vi "Initialize.vi"(8 "error in (no error)":errorcluster, 11 "TelFocus in":refnum<class "TelFocus.lvclass">) -> (0 "error out":errorcluster, 3 "TelFocus out":refnum<class "TelFocus.lvclass">)   [LabVIEW 2018, in "TelFocus.lvclass"]
uses:
  TelFocus.lvclass
  Server/Server.lvclass
  Comm/Stream/Stream.lvclass
  Log/Log.lvclass
  SecMirror/SecMirror.lvclass
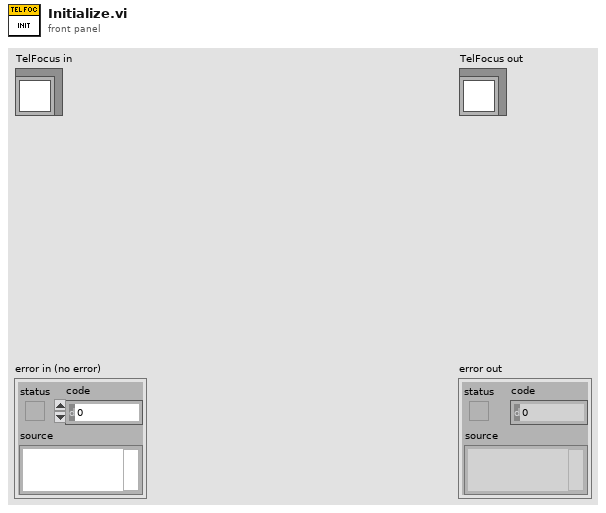
[diagram p1: front panel]
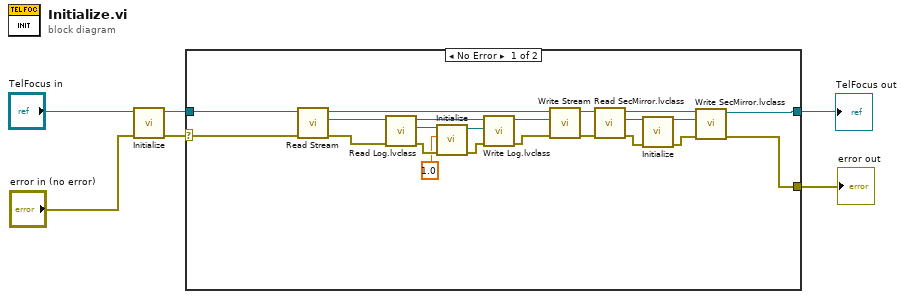
[diagram p0: block diagram]
diagram:
  n1 = call-parent "Initialize.vi"("error in (no error)"="error in (no error)", "Server in"="TelFocus in") -> ("error out"=w3:errorcluster, "Server out"=w4:refnum<class "TelFocus.lvclass">)  [unwired: 8 in]
  n2 = case shown="No Error" w3 {
    selector: w3 -> [w18 w29]
    tunnel: w4 -> [w19 w30]
    tunnel: [w9 w30] -> w2
    tunnel: [w10 w29] -> w1
    frame No Error {
      n3 = call-dynamic "Read Stream.vi"("error in (no error)"=w18, "Server in"=w19) -> ("error out"=w7:errorcluster, "Stream.lvclass"=w8:refnum<class "Stream.lvclass">, "Server out"=w28:refnum<class "TelFocus.lvclass">)  [unwired: 7 in]
      n4 = call-dynamic "Read Log.lvclass.vi"("error in (no error)"=w7, "Comm in"=w8) -> ("error out"=w24:errorcluster, "Log.lvclass"=w26:refnum<class "Log.lvclass">, "Comm out"=w27:refnum<class "Stream.lvclass">)  [unwired: 7 in]
      n5 = call-dynamic "Initialize.vi"("error in (no error)"=w24, "Level"=1.0, "Log in"=w26) -> ("error out"=w23:errorcluster, "Log out"=w25:refnum<class "Log.lvclass">)  [unwired: 7 in]
      n6 = call-dynamic "Write Log.lvclass.vi"("error in (no error)"=w23, "Log.lvclass"=w25, "Comm in"=w27) -> ("error out"=w21:errorcluster, "Comm out"=w22:refnum<class "Stream.lvclass">)  [unwired: 7 in]
      n7 = call-dynamic "Write Stream.vi"("error in (no error)"=w21, "Stream.lvclass"=w22, "Server in"=w28) -> ("error out"=w16:errorcluster, "Server out"=w17:refnum<class "TelFocus.lvclass">)  [unwired: 7 in]
      n8 = call-dynamic "Read SecMirror.lvclass.vi"("error in (no error)"=w16, "TelFocus in"=w17) -> ("error out"=w12:errorcluster, "SecMirror.lvclass"=w15:refnum<class "SecMirror.lvclass">, "TelFocus out"=w13:refnum<class "TelFocus.lvclass">)  [unwired: 7 in]
      n9 = call-dynamic "Initialize.vi"("error in (no error)"=w12, "SecMirror in"=w15) -> ("error out"=w11:errorcluster, "SecMirror out"=w14:refnum<class "SecMirror.lvclass">)  [unwired: 8 in]
      n10 = call-dynamic "Write SecMirror.lvclass.vi"("error in (no error)"=w11, "SecMirror.lvclass"=w14, "TelFocus in"=w13) -> ("error out"=w10:errorcluster, "TelFocus out"=w9:refnum<class "TelFocus.lvclass">)  [unwired: 7 in]
    }
    frame Error {
    }
  }
  "error out" <- w1
  "TelFocus out" <- w2
